vi "Query Alarm Status.vi"(8 "error in (no error)":errorcluster, 11 "2230G in":refnum<class "2230G.lvclass">) -> (0 "error out":errorcluster, 2 "Alarm":bool, 3 "2230G out":refnum<class "2230G.lvclass">)   [LabVIEW 2018, in "2230G.lvlib" / "2230G.lvclass"]
doc: "This Override queries the running status of the power supply's communication session. The 2230G API does not provide for an alarm status. Instead, a system error is queried here, and if true, the status is shown as an existing alarm."
uses:
  2230G.lvclass
  <instrlib>/Keithley KE22xx Series/Keithley KE22xx Series.lvlib
  PPLs/Power Supply/Parent/Power_Supply.lvlibp/Power Supply.lvclass
  C:/Projects/LabVIEW/PPLs/Power Supply/Parent/Power_Supply.lvlibp/Power Supply.lvclass
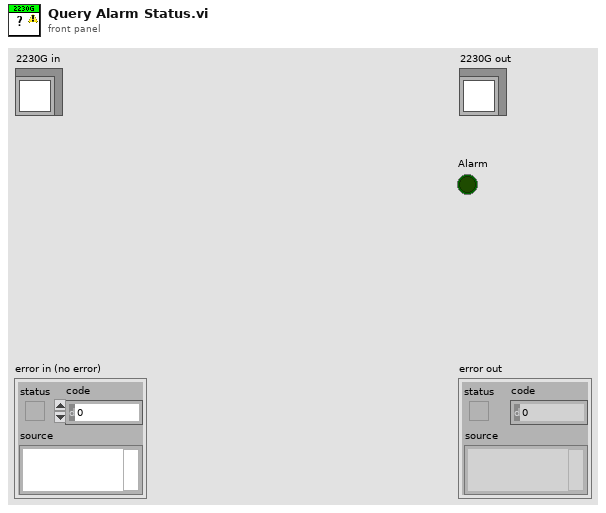
[diagram p1: front panel]
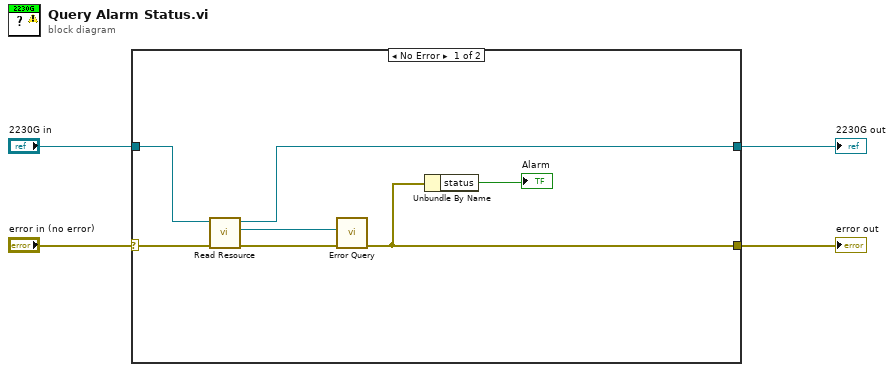
[diagram p0: block diagram]
diagram:
  n1 = case shown="No Error" "error in (no error)" {
    selector: "error in (no error)" -> [w11 w12]
    tunnel: "2230G in" -> [w10 w13]
    tunnel: [w8 w13] -> w2
    tunnel: [w5 w12] -> w1
    frame No Error {
      n2 = call "Read Resource.vi"("error in"=w11, "Power Supply in"=w10) -> ("error out"=w9:errorcluster, "Resource"=w7:refnum<visa-resource-name>, "Power Supply out"=w8:refnum<class "2230G.lvclass">)  [unwired: 7 in]
      n3 = call <instrlib>:"Error Query.vi"("error in (no error)"=w9, "VISA resource name"=w7) -> ("error out"=w5:errorcluster)  [unwired: 6 in, 3 out]
      n4 = Unbundle By Name(w5) -> ("status"=→"Alarm":bool)
    }
    frame Error {
    }
  }
  "error out" <- w1
  "2230G out" <- w2
